vi "Connect.vi"(8 "error in (no error)":errorcluster, 11 "Gen 2 in":refnum<class "Gen 2.lvclass">) -> (0 "error out":errorcluster, 3 "Gen 2 out":refnum<class "Gen 2.lvclass">)   [LabVIEW 2018, in "Gen 2.lvlib" / "Gen 2.lvclass"]
doc: "Connect to Laser over specified VISA Resource"
uses:
  Gen 2.lvclass
  Custom Controls/Serial Settings.ctl
  <vilib>/Instr/_visa.llb/VISA Configure Serial Port (Instr).vi
  PPLs/Laser/Parent/Laser.lvlibp/Laser.lvclass
  C:/Projects/LabVIEW/PPLs/Laser/Parent/Laser.lvlibp/Laser.lvclass
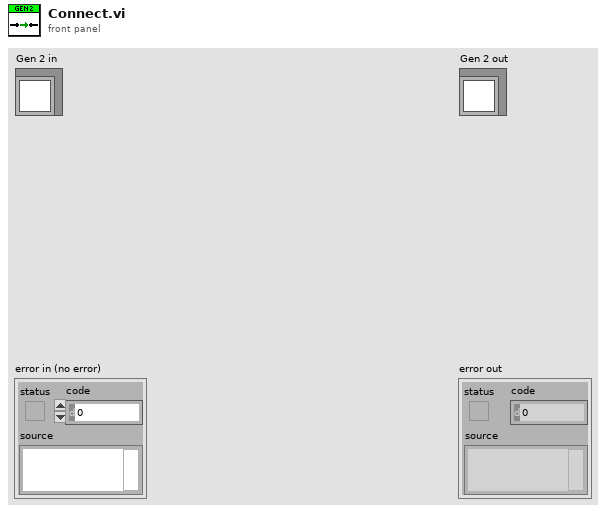
[diagram p1: front panel]
types:
  T1 = typedef "Gen 2.lvlib/Gen 2.lvclass/Serial Settings.ctl" = cluster{"Baud Rate":u32, "Data Bits (8)":u16, "Stop Bits (10: 1 bit)":u16, "Termination Char":bool, "Termination Char (0xA = '\\n' = LF) ":u8, "Parity (0:none)":enum16{"None", "Odd", "Even", "Mark", "Space"}, "Timeout (10sec)":u32, "Flow Control (0:none)":u16}
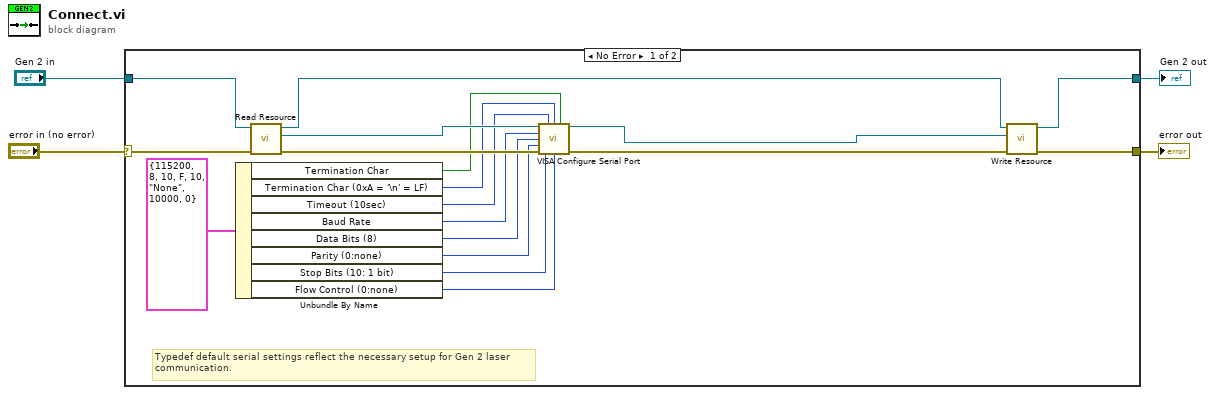
[diagram p0: block diagram]
diagram:
  n1 = case shown="No Error" "error in (no error)" {
    selector: "error in (no error)" -> [w11 w23]
    tunnel: "Gen 2 in" -> [w21 w24]
    tunnel: [w8 w24] -> w3
    tunnel: [w7 w23] -> w2
    frame No Error {
      # "Typedef default serial settings reflect the necessary setup for Gen 2 laser \ncommunication."
      n2 = Unbundle By Name(T1 {"Baud Rate"=115200, "Data Bits (8)"=8, "Stop Bits (10: 1 bit)"=10, "Termination Char"=FALSE, "Termination Char (0xA = '\\n' = LF) "=10, "Parity (0:none)"=enum."None", "Timeout (10sec)"=10000, "Flow Control (0:none)"=0} ("Serial Settings")) -> ("Termination Char"=w10:bool, "Termination Char (0xA = '\\n' = LF)"=w13:u8, "Timeout (10sec)"=w12:u32, "Baud Rate"=w18:u32, "Data Bits (8)"=w17:u16, "Parity (0:none)"=w16:enum16{"None", "Odd", "Even", "Mark", "Space"}, "Stop Bits (10: 1 bit)"=w15:u16, "Flow Control (0:none)"=w14:u16)
      n3 = call "Read Resource.vi"("error in (no error)"=w11, "Laser in"=w21) -> ("error out"=w22:errorcluster, "Resource"=w20:refnum<visa-resource-name>, "Laser out"=w9:refnum<class "Gen 2.lvclass">)  [unwired: 7 in]
      n4 = call-poly "VISA Configure Serial Port"("VISA resource name"=w20, "timeout (10sec)"=w12, "termination char\n(0xA = '\\n' = LF)"=w13, "Enable Termination\nChar (T)"=w10, "baud rate (9600)"=w18, "data bits (8)"=w17, "parity (0:none)"=w16, "error in (no error)"=w22, "stop bits (10: 1 bit)"=w15, "flow control (0:none)"=w14) -> ("VISA resource name out"=w5:refnum<visa-resource-name>, "error out"=w6:errorcluster)  [unwired: 4 in]
      n5 = call "Write Resource.vi"("error in (no error)"=w6, "Resource"=w5, "Laser in"=w9) -> ("error out"=w7:errorcluster, "Laser out"=w8:refnum<class "Gen 2.lvclass">)  [unwired: 7 in]
    }
    frame Error {
    }
  }
  "error out" <- w2
  "Gen 2 out" <- w3
